vi "Get Oneof Template Directory.vi"() -> (0 "appended path":path)   [LabVIEW 2019, in "gRPC Template Creation Utility.lvlib"]
uses:
  gRPC Template Creation Utility.lvlib
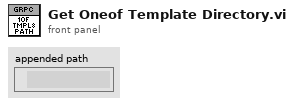
[diagram p1: front panel]
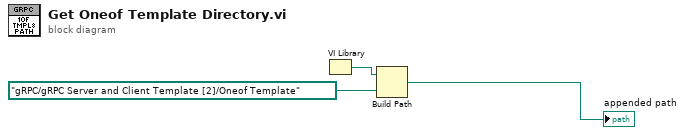
[diagram p0: block diagram]
diagram:
  n1 = VI Library() -> (path=w1:path)
  n2 = Build Path(base path=w1, name or relative path=path "gRPC/gRPC Server and Client Template [2]/Oneof Template") -> (appended path=→"appended path":path)
